vi "sNIST Timesync.vi"(6 "stop":bool, 10 "Minutes to wait":u32=5 min=3, 11 "IP Address of NIST Time Server":string(combo)) -> (0 "NIST Time Failed to Read":bool, 3 "NIST Time":u64)   [LabVIEW 2012]
panel:
  out "Stopped":bool
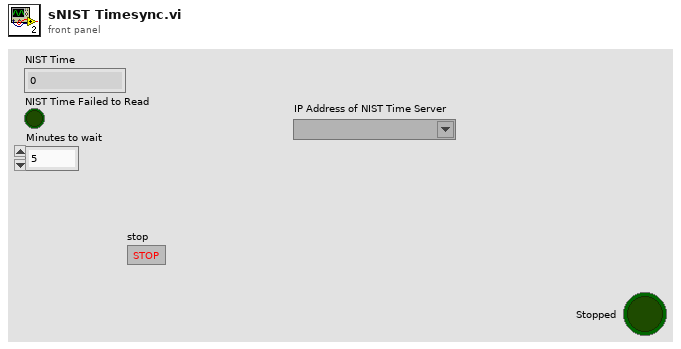
[diagram p1: front panel]
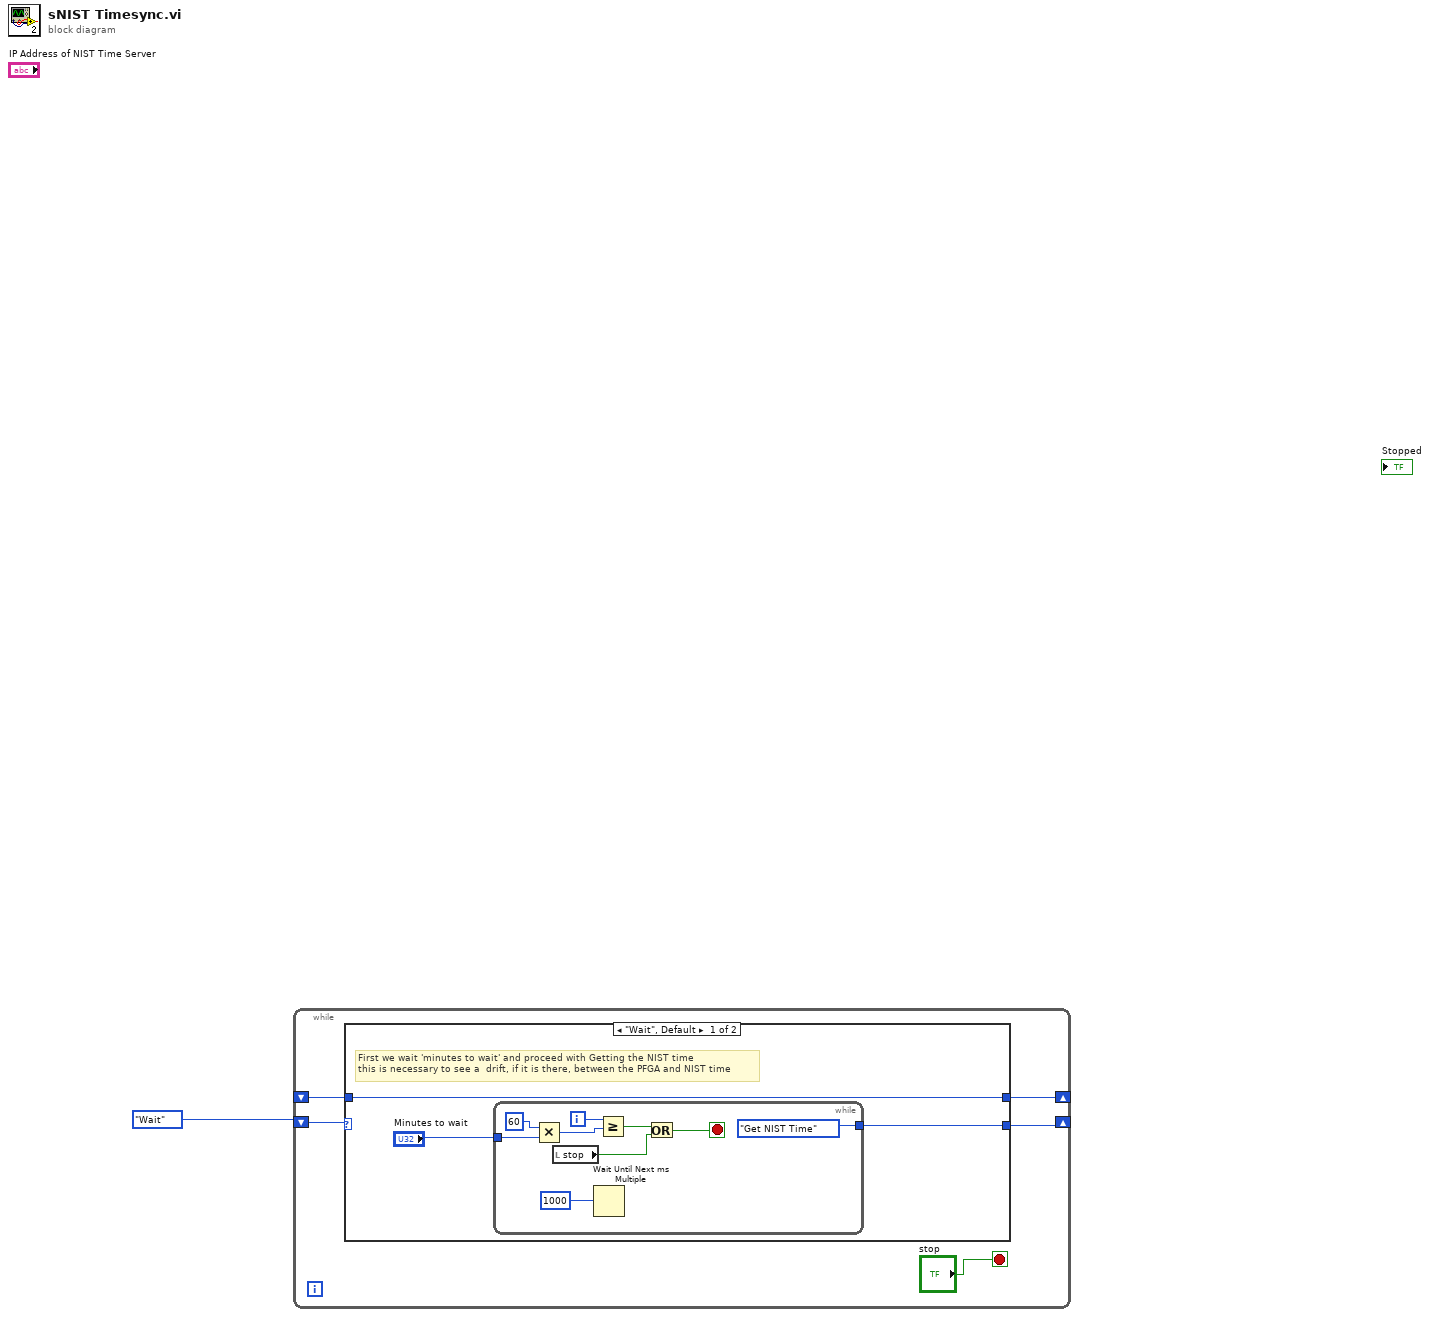
[diagram p0: block diagram]
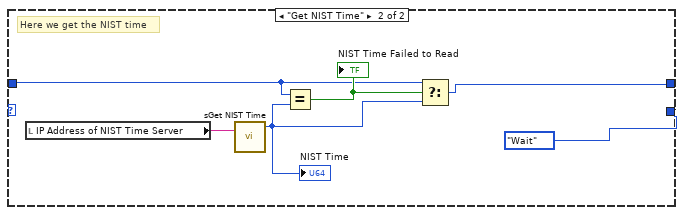
[diagram p2: hidden frame]
diagram:
  n1 = while {
    shift-right: [w5] -> _
    shift-left: enum16{"Wait", "Get NIST Time", "Write"}."Wait" -> [w6]
    shift-right: [w4] -> _
    shift-left: _ -> [w3]
    stop <- "stop" stop-if-true
    n2 = case shown="\"Wait\", Default" w6 {
      tunnel: [w9 enum16{"Wait", "Get NIST Time", "Write"}."Wait"] -> w5
      tunnel: [w8 w24] -> w4
      tunnel: w3 -> [w8 w21]
      frame "Wait", Default {
        # "First we wait 'minutes to wait' and proceed with Getting the NIST time\nthis is necessary to see a  drift, if it is there, between the PFGA and NIST time"
        n3 = while {
          tunnel: [enum16{"Wait", "Get NIST Time", "Write"}."Get NIST Time"] -> w9
          tunnel: "Minutes to wait" -> [w12]
          i -> [w14]
          stop <- w15 stop-if-true
          n4 = Multiply(x=60, y=w12) -> (x*y=w11:u32)
          n5 = local read "stop"() -> (w10:bool)
          n6 = Wait Until Next ms Multiple(millisecond multiple=u32 1000 ("y")) -> ()  [unwired: 1 out]
          n7 = Greater Or Equal?(x=w14, y=w11) -> (x >= y?=w16:bool)
          n8 = Or(x=w16, y=w10) -> (x .or. y?=w15:bool)
        }
      }
      frame "Get NIST Time" {
        # "Here we get the NIST time"
        n9 = local read "IP Address of NIST Time Server"() -> (w19:string)
        n10 = call "sGet NIST Time.vi"("IP Address of NIST Server"=w19) -> ("NTP Time"=w23:u64)  [unwired: 1 in, 2 out]
        "NIST Time" <- w23
        n11 = Equal?(x=w21, y=w23) -> (x = y?=w22:bool)
        "NIST Time Failed to Read" <- w22
        n12 = Select(t=w21, s=w22, f=w23) -> (s? t:f=w24:u64)
      }
    }
  }
